vi "Create.vi"(8 "error in (no error)":errorcluster caption="错误输入（无错误）", 10 "DataGridView":refnum<k24>, 11 "Employee 输入":refnum<class "Employee.lvclass"> caption="DNL_LabVIEW Object in") -> (0 "error out":errorcluster caption="错误输出", 3 "Employee 输出":refnum<class "Employee.lvclass"> caption="DNL_LabVIEW Object out")   [LabVIEW 2012, in "Employee.lvclass"]
uses:
  Employee.lvclass
  System.Windows.Forms
  Employee.lvclass/Employee.ctl
  Data Set/DataSet.lvclass
  Data Table/DataTable.lvclass
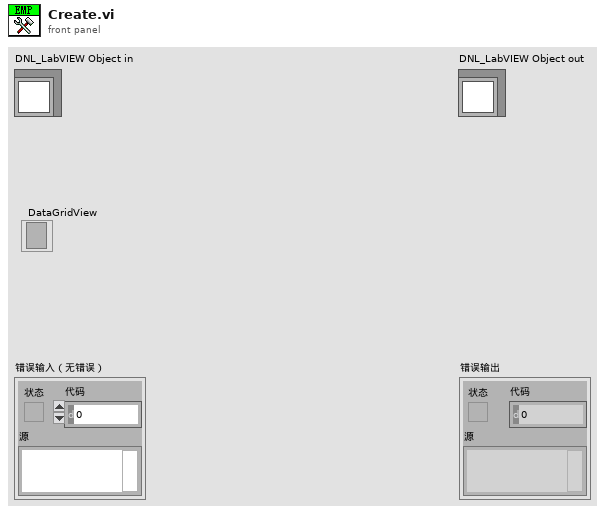
[diagram p1: front panel]
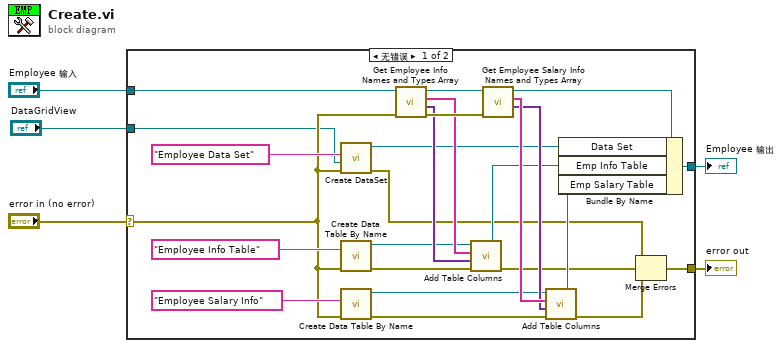
[diagram p0: block diagram]
diagram:
  n1 = case shown="无错误" "error in (no error)" {
    selector: "error in (no error)" -> [w7 w32]
    tunnel: [w21 w32] -> w4
    tunnel: [w22 w31] -> w2
    tunnel: "Employee 输入" -> [w30 w31]
    tunnel: "DataGridView" -> [w6 _]
    frame No Error {
      n2 = call "Create DataSet.vi"("error in (no error)"=w7, "DataGridView"=w6, "dataSetName"="Employee Data Set") -> ("error out"=w11:errorcluster, "DataSet 输出"=w19:refnum<class "DataSet.lvclass">)  [unwired: 7 in]
      n3 = call "Create Data Table By Name.vi"("error in (no error)"=w7, "tableName"="Employee Info Table") -> ("error out"=w10:errorcluster, "DataTable 输出"=w17:refnum<class "DataTable.lvclass">)  [unwired: 8 in]
      n4 = call "Create Data Table By Name.vi"("error in (no error)"=w7, "tableName"="Employee Salary Info") -> ("error out"=w9:errorcluster, "DataTable 输出"=w8:refnum<class "DataTable.lvclass">)  [unwired: 8 in]
      n5 = call "Get Employee Info Names and Types Array.vi"("error in (no error)"=w7, "Employee 输入"=w30) -> ("error out"=w28:errorcluster, "Colomn Types"=w25:variant[], "Column Names"=w26:string[], "Employee 输出"=w29:refnum<class "Employee.lvclass">)  [unwired: 6 in]
      n6 = call "Add Table Columns.vi"("error in (no error)"=w10, "DataColunm Types"=w25, "DataColumn Names"=w26, "DataTable 输入"=w17) -> ("error out"=w13:errorcluster, "DataTable 输出"=w16:refnum<class "DataTable.lvclass">)  [unwired: 6 in]
      n7 = call "Get Employee Salary Info Names and Types Array.vi"("error in (no error)"=w28, "Employee 输入"=w29) -> ("Colomn Types"=w23:variant[], "Column Names"=w24:string[], "Employee 输出"=w27:refnum<class "Employee.lvclass">)  [unwired: 6 in, 1 out]
      n8 = call "Add Table Columns.vi"("error in (no error)"=w9, "DataColunm Types"=w23, "DataColumn Names"=w24, "DataTable 输入"=w8) -> ("error out"=w12:errorcluster, "DataTable 输出"=w14:refnum<class "DataTable.lvclass">)  [unwired: 6 in]
      n9 = Bundle By Name(cluster=w27, "Data Set"=w19, "Emp Info Table"=w16, "Emp Salary Table"=w14) -> (w22:refnum<class "Employee.lvclass">)
      n10 = Merge Errors(w11, w13, w12) -> (w21:errorcluster)
    }
    frame Error {
    }
  }
  "error out" <- w4
  "Employee 输出" <- w2
